vi "Chebybezier2.vi"(9 "Numeric":dbl, 10 "order":u32, 11 "Y":sgl[][](array[numeric])) -> (3 "C":dbl[](array[numeric]) format="%.2f")   [LabVIEW 2019]
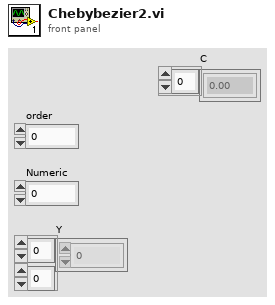
[diagram p1: front panel]
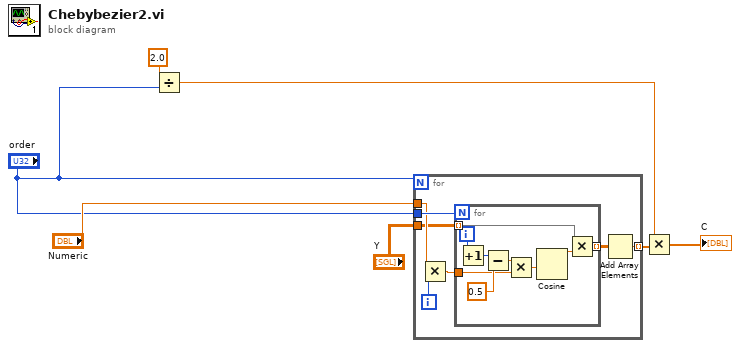
[diagram p0: block diagram]
diagram:
  n1 = Divide(x=2.0, y="order") -> (x/y=w1:dbl)
  n2 = for {
    N: "order" -> [_]
    tunnel: "order" -> [w14]
    tunnel: "Numeric" -> [w13]
    tunnel: "Y" -> [w11]
    tunnel: [w9] -> w6 mode=indexing
    i -> [w8]
    n3 = Multiply(x=w13, y=w8) -> (x*y=w12:dbl)
    n4 = for {
      N: w14 -> [_]
      tunnel: w12 -> [w15]
      tunnel: w11 -> [w22] mode=indexing
      tunnel: [w21] -> w10 mode=indexing
      i -> [w20]
      n5 = Increment(x=w20) -> (x+1=w16:i32)
      n6 = Subtract(x=w16, y=0.5) -> (x-y=w18:dbl)
      n7 = Multiply(x=w18, y=w15) -> (x*y=w17:dbl)
      n8 = Cosine(x=w17) -> (cos(x)=w23:dbl)
      n9 = Multiply(x=w22, y=w23) -> (x*y=w21:dbl[])
    }
    n10 = Add Array Elements(numeric array=w10) -> (sum=w9:dbl)
  }
  n11 = Multiply(x=w1, y=w6) -> (x*y=→"C":dbl[])
